vi "Next Capture (Greyscale).vi"(8 "error in (no error)":errorcluster, 9 "Timeout (Default: 1000 ms)":u16=1000 format="%.0f ms", 10 "Greyscale Destination Image in":T1, 11 "Stream in":refnum<class "Stream.lvclass">) -> (0 "error out":errorcluster, 1 "Timed Out?":bool, 2 "Greyscale Destination Image":T1, 3 "Stream":refnum<class "Stream.lvclass">)   [LabVIEW 2020, in "capture.lvlib" / "Stream.lvclass"]
doc: "Wait for the Next Capture to be copied into the Image Destination."
uses:
  Stream.lvclass
  image/Greyscale Image.ctl
  Stream.lvclass/Stream.ctl
  66171ef0-1d22-3fc5-88a4-b174a611e83f.vi
  <vilib>/Utility/error.llb/Error Cluster From Error Code.vi
  image/image.lvlib
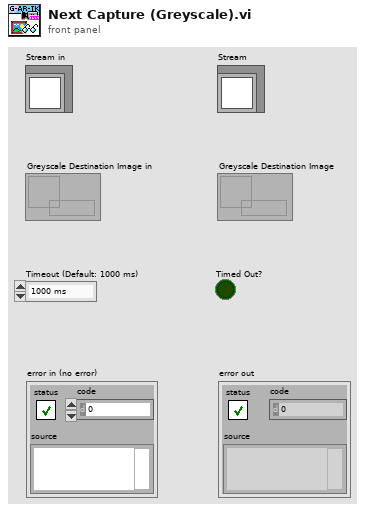
[diagram p1: front panel]
types:
  T1 = typedef "image.lvlib/Greyscale Image.ctl" = refnum<data-value>
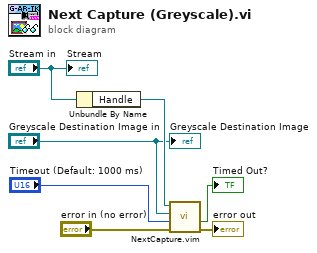
[diagram p0: block diagram]
diagram:
  n1 = Unbundle By Name("Stream in") -> ("Handle"=w7:refnum<data-value>)
  n2 = call "NextCapture.vim"("error in (no error)"="error in (no error)", "Timeout (Default: 1000 ms)"="Timeout (Default: 1000 ms)", "ARGB Image Destination in"="Greyscale Destination Image in", "Handle"=w7) -> ("error out"=→"error out":errorcluster, "Timed Out?"=→"Timed Out?":bool)  [unwired: 6 in]
  "Stream" <- "Stream in"
  "Greyscale Destination Image" <- "Greyscale Destination Image in"
